vi "Create.vi"(8 "error in":errorcluster, 11 "IUnmanaged in":refnum<class "IUnmanaged.lvclass">) -> (0 "error out":errorcluster, 3 "IUnmanaged out":refnum<class "IUnmanaged.lvclass">)   [LabVIEW 2025, in "IUnmanaged.lvclass"]
uses:
  IUnmanaged.lvclass
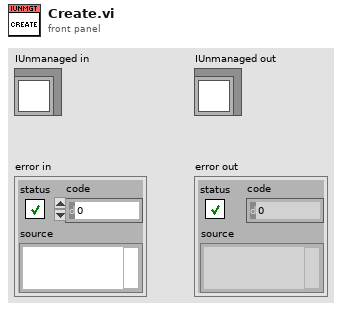
[diagram p1: front panel]
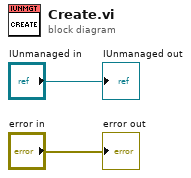
[diagram p0: block diagram]
diagram:
  "error out" <- "error in"
  "IUnmanaged out" <- "IUnmanaged in"
